vi "SP Interpolate Attenuation Values.vi"(4 "Instance (First)":enum16{"First", "Last"}(ring), 6 "Attenuation Value":dbl, 8 "X Values":dbl[](array[numeric]), 9 "Y Values":dbl[](array[numeric])) -> (1 "Interpolated X Value":dbl)   [LabVIEW 2011]
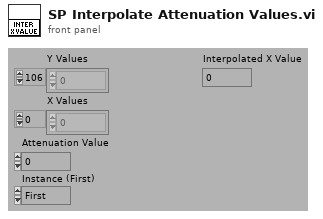
[diagram p1: front panel]
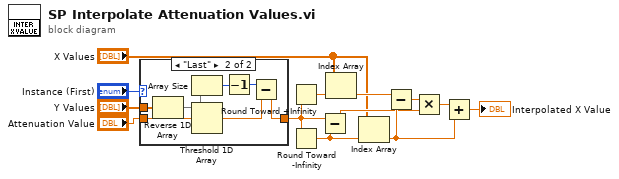
[diagram p0: block diagram]
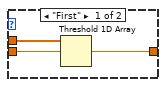
[diagram p2: hidden frame]
diagram:
  n1 = case shown="\"Last\"" "Instance (First)" {
    tunnel: [w15 w17] -> w9
    tunnel: "Attenuation Value" -> [w14 w23]
    tunnel: "Y Values" -> [w16 w22]
    frame "First" {
      n2 = Threshold 1D Array(2:w14, 3:w16) -> (0:w15:dbl)  [unwired: 1 out]
    }
    frame "Last" {
      n3 = Reverse 1D Array(array=w22) -> (reversed array=w21:dbl[])
      n4 = Array Size(array=w21) -> (size(s)=w20:i32)
      n5 = Threshold 1D Array(2:w23, 3:w21) -> (0:w18:dbl)  [unwired: 1 out]
      n6 = Decrement(x=w20) -> (x-1=w19:i32)
      n7 = Subtract(x=w19, y=w18) -> (x-y=w17:dbl)
    }
  }
  n8 = Round Toward +Infinity(x=w9) -> (ceil(x): smallest int >= x=w8:dbl)
  n9 = Round Toward -Infinity(1:w9) -> (0:w7:dbl)
  n10 = Subtract(x=w9, y=w7) -> (x-y=w6:dbl)
  n11 = Index Array(array="X Values", index=w8) -> (element=w13:dbl)
  n12 = Index Array(array="X Values", index=w7) -> (element=w12:dbl)
  n13 = Subtract(x=w13, y=w12) -> (x-y=w11:dbl)
  n14 = Multiply(x=w11, y=w6) -> (x*y=w10:dbl)
  n15 = Add(x=w10, y=w12) -> (x+y=→"Interpolated X Value":dbl)
